vi "Write Ramp Volt.vi"(8 "error in":errorcluster, 10 "Voltage_Ramp":dbl, 11 "69X_79X in":refnum<class "7976A.lvclass">) -> (0 "error out":errorcluster, 3 "69X_79X out":refnum<class "7976A.lvclass">)   [LabVIEW 2019, in "7976A.lvlib" / "7976A.lvclass"]
uses:
  Library/7976A.lvclass
  C:/Users/Public/Documents/Development/builds/Instruments/PowerSupply.lvlibp/Library/PowerSupply.lvclass
  builds/Instruments/PowerSupply.lvlibp/Library/PowerSupply.lvclass
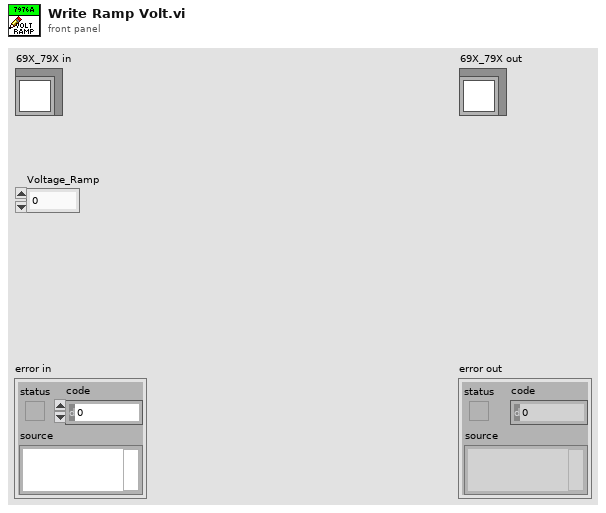
[diagram p1: front panel]
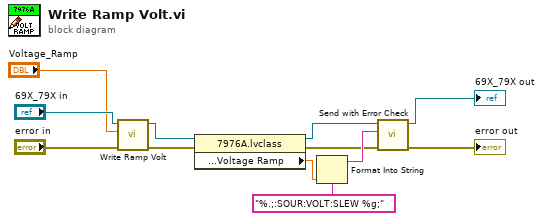
[diagram p0: block diagram]
diagram:
  n1 = call-parent "Write Ramp Volt.vi"("error in"="error in", "Voltage_Ramp"="Voltage_Ramp", "PowerSupply in"="69X_79X in") -> ("error out"=w10:errorcluster, "PowerSupply out"=w3:refnum<class "7976A.lvclass">)  [unwired: 7 in]
  n2 = property class="7976A.lvclass"(reference=w3, error in=w10) -> (reference out=w2:refnum<class "7976A.lvclass">, error out=w4:errorcluster, "Accessors:Setting:Ramp:Voltage Ramp"=w1:dbl)
  n3 = Format Into String(format string="%.;:SOUR:VOLT:SLEW %g;", w1) -> (resulting string=w9:string)  [unwired: 2 in, 1 out]
  n4 = call "Send with Error Check.vi"("error in (no error)"=w4, "Command"=w9, "7976A in"=w2) -> ("error out"=→"error out":errorcluster, "7976A out"=→"69X_79X out":refnum<class "7976A.lvclass">)  [unwired: 7 in]
